vi "createTitles-FRA.vi"(9 "Sensor Number":i32) -> (3 "String":string)   [LabVIEW 2014]
doc: "André Romero - 2017\nandretec@ifsc.usp.br"
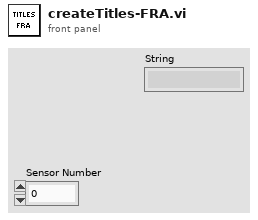
[diagram p1: front panel]
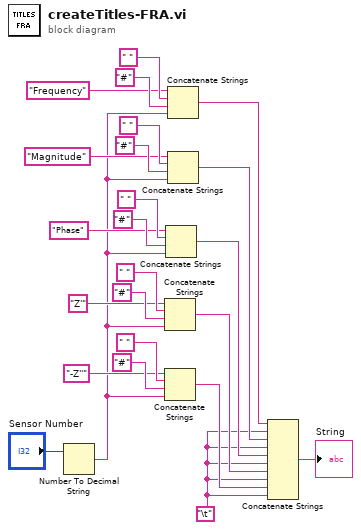
[diagram p0: block diagram]
diagram:
  w1 = "\t"
  n1 = Number To Decimal String(number="Sensor Number") -> (decimal integer string=w5:string)  [unwired: 1 in]
  n2 = Concatenate Strings("Z'" ("string"), " " ("string"), "#" ("string"), w5) -> (w3:string)
  n3 = Concatenate Strings("-Z''" ("string"), " " ("string"), "#" ("string"), w5) -> (w2:string)
  n4 = Concatenate Strings("Phase" ("string"), " " ("string"), "#" ("string"), w5) -> (w4:string)
  n5 = Concatenate Strings("Frequency" ("string"), " " ("string"), "#" ("string"), w5) -> (w20:string)
  n6 = Concatenate Strings("Magnitude" ("string"), " " ("string"), "#" ("string"), w5) -> (w23:string)
  n7 = Concatenate Strings(w20, w1, w23, w1, w4, w1, w3, w1, w2, w1) -> (→"String":string)
